vi "RootBLE.vi"() -> ()   [LabVIEW 2019]
uses:
  <userlib>/MicroPython/VIs/uPythonX/uPythonX.xctl
panel:
  in  "PyBD 3":T1(xcontrol)={"Port"="pyboard - ASRL96::INSTR", "All Code"="import bluetooth, machine, utime,ubinascii\n\ndef ble_cb(event, data):\n     global bt_event,bt_data,devices\n     bt_event = event, data\n     print('ble event:', event, data)\n     \nbt = bluetooth.Bluetooth()\nbt.active(1)\nbt_event=None\nbt.irq(ble_cb, 0xffff)\n\ndef sync_cmd(f, args, timeout_ms=1000):\n    global bt_event\n    event = []\n    bt_event = None # clear event\n    f(*args) # call function\n    t0 = utime.ticks_ms()\n    while time.ticks_diff(time.ticks_ms(), t0) < timeout_ms:\n        if bt_event is not None:\n             event.append(bt_event)\n             bt_event = None\n        machine.idle() \n    return event\n    #raise OSError('timeout')\n\n# use it like this\nread_result = sync_cmd(bt.scan, (5000), 5000)\nfor i in read_result:\n     print('Addr type: %d mac addr: %s'%(i[1][0],ubinascii.hexlify(i[1][1],':')))\n\nsync_cmd(bt.connect,(1,b'\\x34\\x15\\x13\\x7F\\xD5\\xCC'))\n\n#bt.connect(2,b'\\x34\\x15\\x13\\x7F\\xD5\\xCC')"}
  in  "VISA resource name":refnum<visa-resource-name>
  in  "PyBD 2":T1(xcontrol)={"Port"="PyBoard - ASRL44::INSTR", "All Code"="import bluetooth, machine, utime\n\nbt_event = 0,0\nbt_data = []\ndevices = []\n\ndef ble_cb(event, data):\n     global bt_event,bt_data,devices\n     bt_event = event, data\n     if event == 16:\n          devices.append(data)\n     else:\n          bt_data.append(bt_event)\n     print('ble event:', event, data)\n          \n\nbt = bluetooth.Bluetooth()\nbt.active(1)\nbt_event=None\nbt.irq(ble_cb, 0xffff)\n\n\nbt.connect(1,b'\\xf6\\x1d\\xa5\\xe2^\\xf5')\n\nbt.disconnect(64)\n\nwhile not bt_event:\n     machine.idle()\n\nbt.gattc_write(14, 64, b'\\x01')\n\n'''\nThen the available functions for central mode are:\n\nbt.connect(addr_type, mac, scan_duration_ms=2000)\nbt.scan(duration_ms)\nbt.gattc_disc_svcs(conn_handle)\nbt.gattc_disc_chrs(start_handle, end_handle, conn_handle)\nbt.gattc_disc_dscs(start_handle, end_handle, conn_handle)\nbt.gattc_read(value_handle, conn_handle)\nbt.gattc_write(value_handle, conn_handle, data)\n\nUsually conn_handle would be 64.  addr_type should probably be 0 (or maybe 2).  mac should be the MAC address of the root robot, which can be found by doing a scan (results come in through the ble_cb callback).\n\nYou then need to find the value handles for the tx/rx characteristics on the root robot.  This is done using: bt.gattc_disc_chrs(0, 0xffff, 64).  ble_cb will then be called with the results of this discovery process and the returned data will include the tx/rx uuid along with the value handle for it (but I'm not sure exactly of the format of the returned data for this...).\n\n'''\nbt_data = []\ndevices = []\nstarttime = utime.time()\nbt.scan(5000)\nwhile (utime.time()- starttime) < 5:\n     bt_event=None\n     while not bt_event:\n          machine.idle()\n     \n\nbt.connect(0, b'M\\x0b\\xf0\\xf9\\x81\\x00')\n\n# ble event: 16 (1, b'\\xf6\\x1d\\xa5\\xe2^\\xf5', True, 198, b'\\x02\\x01\\x06\\x11\\x06yI\\xb0\"\\x98\\x0c\\xa3\\x97-D*\\xac(\\xd8\\xc5H')\nbt.connect(1,b'\\xf6\\x1d\\xa5\\xe2^\\xf5')\n#ble event: 64 (1, b'\\xf6\\x1d\\xa5\\xe2^\\xf5', 64)\nbt.gattc_disc_svcs(64)\n'''\nble event: 256 (1, 7, UUID16(0x1800), 64)\nble event: 256 (8, 8, UUID16(0x1801), 64)\nble event: 256 (9, 14, UUID128('6e400001-b5a3-f393-e0a9-e50e24dcca9e'), 64)\nble event: 256 (15, 30, UUID16(0x180a), 64)\nble event: 256 (31, 65535, UUID128('48c5d828-ac2a-442d-97a3-0c9822b04979'), 64)\n     \nble event: 256 (64, 1, 7, UUID16(0x1800))\nble event: 256 (64, 8, 8, UUID16(0x1801))\nble event: 256 (64, 9, 14, UUID128('9ecadc24-0ee5-a9e0-93f3a3b50100406e')) # uart_identifier_uuid\nble event: 256 (64, 15, 30, UUID16(0x180a))\nble event: 256 (64, 31, 65535, UUID128('7949b022-980c-a397-2d442aac28d8c548'))  # root_identifier_uuid - backwards\n'''\n#bt.gattc_discover_characteristics(64, 9, 14)\n\n\nbt.gattc_disc_chrs(9,14,64)\nbt.gattc_disc_chrs(1,7,64)\nbt.gattc_read(3,64)   # get name\nbt.gattc_disc_dscs(1, 65535, 64)\nbt.gattc_write(14, 64, b'\\x01')\n\ndef get_name (data):\n     bt.connect(data[0],data[1])\n     bt.data=[]\n     whilin\n     bt.gattc_disc_svcs(64)\n     bt.gattc_disc_chrs(9,14,64)\n     \n\n'''\n1. get listing of all BT devices\n2. connect to each and\n3. ask for all servies\n4. find service 0x1800 - discover characteristics\n5. do a read of the characterstic for 0x2A00\n6. take the last (3rd) element - that is the name\n7. disconnect\n'''\nble event: 512 (10, 11, 12, UUID128('6e400002-b5a3-f393-e0a9-e50e24dcca9e'), 64)\nble event: 512 (12, 13, 16, UUID128('6e400003-b5a3-f393-e0a9-e50e24dcca9e'), 64)\n     \n\nble event: 512 (64, 10, 11, 12, UUID128('9ecadc24-0ee5-a9e0-93f3a3b50200406e'))   #  tx characteristic\nble event: 512 (64, 12, 13, 16, UUID128('9ecadc24-0ee5-a9e0-93f3a3b50300406e'))   #  rx characteristic\n'''\nforward = [0x01, 0x04, 0x00, 0x00, 0x00, 0x00, 0x64, 0x00, 0x00, 0x00, 0x64, 0x00, 0x00, 0x00, 0x00, 0x00, 0x00, 0x00, 0x00, 0xD1]\nleft = [0x01, 0x04, 0x00, 0x00, 0x00, 0x00, 0x00, 0x00, 0x00, 0x00, 0x64, 0x00, 0x00, 0x00, 0x00, 0x00, 0x00, 0x00, 0x00, 0x8A]\nright = [0x01, 0x04, 0x00, 0x00, 0x00, 0x00, 0x64, 0x00, 0x00, 0x00, 0x00, 0x00, 0x00, 0x00, 0x00, 0x00, 0x00, 0x00, 0x00, 0x25]\nstop = [0x01, 0x04, 0x00, 0x00, 0x00, 0x00, 0x00, 0x00, 0x00, 0x00, 0x00, 0x00, 0x00, 0x00, 0x00, 0x00, 0x00, 0x00, 0x00, 0x7E]\nbackwards = [0x01, 0x04, 0x00, 0xFF, 0xFF, 0xFF, 0x9C, 0xFF, 0xFF, 0xFF, 0x9C, 0x00, 0x00, 0x00, 0x00, 0x00, 0x00, 0x00, 0x00, 0x71]\npen_up = [0x02, 0x00, 0x00, 0x00, 0x00, 0x00, 0x00, 0x00, 0x00, 0x00, 0x00, 0x00, 0x00, 0x00, 0x00, 0x00, 0x00, 0x00, 0x00, 0x00]\npen_down = [0x02, 0x00, 0x00, 0x01, 0x00, 0x00, 0x00, 0x00, 0x00, 0x00, 0x00, 0x00, 0x00, 0x00, 0x00, 0x00, 0x00, 0x00, 0x00, 0x00]\n\nbt.gattc_write(11, 64, bytearray(pen_down))\n\n\n\nbt.gattc_read(16,64)\n# ble event: 2048 (16, 64, b'\\x02\\x11\\x00%*')\n\nbt.disconnect(64)\n\n\ndef TranslateMessage(data):\n     type = ''\n     if event == 2048:\n          message = data[2][0]\n          if message == 4:\n               type = 'Color Sensor'\n          elif message == 12:\n               type = 'Bumper'\n          elif message == 13:\n               type = 'Light Sensor'\n          elif message == 17:\n               type = 'Touch Sensor'\n          elif message == 20:\n               type = 'Cliff Sensor'\n          print(type, message)\n          return data\n          \n'''\n\u0016ble event: 8192 (13, 64, b'\\x11\\x00\\x00\\x00\\x03\\x1dC@\\x00\\x00\\x00\\x00\\x00\\x00\\x00\\x00\\x00\\x00\\x00\\x17')\nble event: 8192 (13, 64, b'\\x11\\x00\\x01\\x00\\x03\\x1d\\xd9\\x00\\x00\\x00\\x00\\x00\\x00\\x00\\x00\\x00\\x00\\x00\\x00!')\nble event: 8192 (13, 64, b'\\r\\x00\\x02\\x00\\x03\\x1e\\xd4\\x06\\x02\\x13\\x00\\x7f\\x00\\x00\\x00\\x00\\x00\\x00\\x00d')\nble event: 8192 (13, 64, b'\\x11\\x00\\x03\\x00\\x03$\\x19@\\x00\\x00\\x00\\x00\\x00\\x00\\x00\\x00\\x00\\x00\\x00D')\nble event: 8192 (13, 64, b'\\x11\\x00\\x04\\x00\\x03%w\\x00\\x00\\x00\\x00\\x00\\x00\\x00\\x00\\x00\\x00\\x00\\x00f')\nble event: 8192 (13, 64, b'\\x0c\\x00\\x05\\x00\\x03*#@\\x00\\x00\\x00\\x00\\x00\\x00\\x00\\x00\\x00\\x00\\x00y')\nble event: 8192 (13, 64, b'\\x0c\\x00\\x06\\x00\\x03+\\x9a\\x00\\x00\\x00\\x00\\x00\\x00\\x00\\x00\\x00\\x00\\x00\\x00\\xf3')\nble event: 8192 (13, 64, b'\\x0c\\x00\\x07\\x00\\x031|\\x80\\x00\\x00\\x00\\x00\\x00\\x00\\x00\\x00\\x00\\x00\\x00\\xb8')\nble event: 8192 (13, 64, b'\\x0c\\x00\\x08\\x00\\x036\\x91\\x00\\x00\\x00\\x00\\x00\\x00\\x00\\x00\\x00\\x00\\x00\\x00\\x9f')\nble event: 8192 (13, 64, b'\\x11\\x00\\t\\x00\\x03A\\x87\\x80\\x00\\x00\\x00\\x00\\x00\\x00\\x00\\x00\\x00\\x00\\x00g')\nble event: 8192 (13, 64, b'\\x11\\x00\\n\\x00\\x03C\\xdf\\x00\\x00\\x00\\x00\\x00\\x00\\x00\\x00\\x00\\x00\\x00\\x00\\xca')\nble event: 8192 (13, 64, b'\\x11\\x00\\x0b\\x00\\x03DC\\x80\\x00\\x00\\x00\\x00\\x00\\x00\\x00\\x00\\x00\\x00\\x00W')\nble event: 8192 (13, 64, b'\\x11\\x00\\x0c\\x00\\x03D\\xd9\\x00\\x00\\x00\\x00\\x00\\x00\\x00\\x00\\x00\\x00\\x00\\x00*')\nble event: 8192 (13, 64, b'\\x11\\x00\\r\\x00\\x03H]@\\x00\\x00\\x00\\x00\\x00\\x00\\x00\\x00\\x00\\x00\\x00\\x0e')\nble event: 8192 (13, 64, b'\\x11\\x00\\x0e\\x00\\x03IW\\x00\\x00\\x00\\x00\\x00\\x00\\x00\\x00\\x00\\x00\\x00\\x00O')\nble event: 8192 (13, 64, b'\\x11\\x00\\x0f\\x00\\x03K\\xe1 \\x00\\x00\\x00\\x00\\x00\\x00\\x00\\x00\\x00\\x00\\x00\\x1c')\nble event: 8192 (13, 64, b'\\x11\\x00\\x10\\x00\\x03Lw\\x00\\x00\\x00\\x00\\x00\\x00\\x00\\x00\\x00\\x00\\x00\\x00}')\nble event: 8192 (13, 64, b'\\x14\\x00\\x11\\x00\\x03m\\xfc\\x01\\x00.\\x001\\x00\\x00\\x00\\x00\\x00\\x00\\x00\\x87')\nble event: 8192 (13, 64, b'\\r\\x00\\x12\\x00\\x03|~\\x06\\x01\\xb2\\x00x\\x00\\x00\\x00\\x00\\x00\\x00\\x00Q')\n     '''"}
  in  "Pi":T1(xcontrol)={"Port"="Spike - ASRL73::INSTR", "All Code"="#!/usr/bin/env python3\n# https://github.com/zlite/PyRoot/blob/master/drive-root.py\n\nimport gatt\nimport threading\nimport time,termios,tty,sys\n\ninstructions = \"\"\"---------------------\n KEY         COMMAND\n---------------------\n w           Forward\n s           Backward\n a           Left\n d           Right\n space       Stop\n t           Turn\n o           Pen Up\n l           Pen Down\n q           Quit\"\"\"\n\n# BLE UUID's\nroot_identifier_uuid = '48c5d828-ac2a-442d-97a3-0c9822b04979'\nuart_service_uuid = '6e400001-b5a3-f393-e0a9-e50e24dcca9e'\ntx_characteristic_uuid = '6e400002-b5a3-f393-e0a9-e50e24dcca9e' # Write\nrx_characteristic_uuid = '6e400003-b5a3-f393-e0a9-e50e24dcca9e' # Notify\n\nclass BluetoothDeviceManager(gatt.DeviceManager):\n    robot = None # root robot device\n\n    def device_discovered(self, device):\n        print(\"[%s] Discovered: %s\" % (device.mac_address, device.alias()))\n        self.stop_discovery() # Stop searching\n        self.robot = RootDevice(mac_address=device.mac_address, manager=self)\n        self.robot.connect()\n\nclass RootDevice(gatt.Device):\n    def connect_succeeded(self):\n        super().connect_succeeded()\n        print(\"[%s] Connected\" % (self.mac_address))\n\n    def connect_failed(self, error):\n        super().connect_failed(error)\n        print(\"[%s] Connection failed: %s\" % (self.mac_address, str(error)))\n\n    def disconnect_succeeded(self):\n        super().disconnect_succeeded()\n        print(\"[%s] Disconnected\" % (self.mac_address))\n\n    def services_resolved(self):\n        super().services_resolved()\n        print(\"[%s] Resolved services\" % (self.mac_address))\n\n        self.uart_service = next(\n            s for s in self.services\n            if s.uuid == uart_service_uuid)\n\n        self.tx_characteristic = next(\n            c for c in self.uart_service.characteristics\n            if c.uuid == tx_characteristic_uuid)\n\n        self.rx_characteristic = next(\n            c for c in self.uart_service.characteristics\n            if c.uuid == rx_characteristic_uuid)\n\n        self.rx_characteristic.enable_notifications() # listen to RX messages\n\n    def characteristic_value_updated(self, characteristic, value):\n        message = []\n        type = \"\"\n        for byte in value:\n            message.append(byte)\n#        print (\"Messages from Root:\")\n        if message[0] == 4: type = \"Color Sensor\"\n        if message[0] == 12: type = \"Bumper\"\n        if message[0] == 13: type = \"Light Sensor\"\n        if message[0] == 17: type = \"Touch Sensor\"\n        if message[0] == 20: type = \"Cliff Sensor\"\n\n        print(type, message)\n\n    def drive_forward(self):\n        self.tx_characteristic.write_value([0x01, 0x04, 0x00, 0x00, 0x00, 0x00, 0x64, \n0x00, 0x00, 0x00, 0x64, 0x00, 0x00, 0x00, 0x00, 0x00, 0x00, 0x00, 0x00, 0xD1])\n\n    def drive_left(self):\n        self.tx_characteristic.write_value([0x01, 0x04, 0x00, 0x00, 0x00, 0x00, 0x00, 0x00, 0x00, 0x00, 0x64, 0x00, 0x00, 0x00, 0x00, 0x00, 0x00, 0x00, 0x00, 0x8A])\n\n    def drive_right(self):\n        self.tx_characteristic.write_value([0x01, 0x04, 0x00, 0x00, 0x00, 0x00, 0x64, 0x00, 0x00, 0x00, 0x00, 0x00, 0x00, 0x00, 0x00, 0x00, 0x00, 0x00, 0x00, 0x25])\n\n    def stop(self):\n        self.tx_characteristic.write_value([0x01, 0x04, 0x00, 0x00, 0x00, 0x00, 0x00, 0x00, 0x00, 0x00, 0x00, 0x00, 0x00, 0x00, 0x00, 0x00, 0x00, 0x00, 0x00, 0x7E])\n\n    def drive_backwards(self):\n        self.tx_characteristic.write_value([0x01, 0x04, 0x00, 0xFF, 0xFF, 0xFF, 0x9C, 0xFF, 0xFF, 0xFF, 0x9C, 0x00, 0x00, 0x00, 0x00, 0x00, 0x00, 0x00, 0x00, 0x71])\n\n    def pen_up(self):\n        self.tx_characteristic.write_value([0x02, 0x00, 0x00, 0x00, 0x00, 0x00, 0x00, 0x00, 0x00, 0x00, 0x00, 0x00, 0x00, 0x00, 0x00, 0x00, 0x00, 0x00, 0x00, 0x00])\n\n    def pen_down(self):\n        self.tx_characteristic.write_value([0x02, 0x00, 0x00, 0x01, 0x00, 0x00, 0x00, 0x00, 0x00, 0x00, 0x00, 0x00, 0x00, 0x00, 0x00, 0x00, 0x00, 0x00, 0x00, 0x00])\n\n    def turn_rate(self, rate):\n        left = 0\n        right = 0\n        if rate >= 0:\n            left = rate\n        if rate < 0:\n            right = -1*rate\n        leftbytes = left.to_bytes(4,byteorder='big',signed=True)  # need to convert to byte string\n        rightbytes = right.to_bytes(4,byteorder='big',signed=True)\n        # note that we're not dynamically calculating the CRC at the end, so just leaving it 0 (unchecked)\n        self.tx_characteristic.write_value([0x01, 0x04, 0x00, leftbytes[0], leftbytes[1], leftbytes[2], leftbytes[3], rightbytes[0], rightbytes[1], rightbytes[2], rightbytes[3], 0x00, 0x00, 0x00, 0x00, 0x00, 0x00, 0x00, 0x00, 0x0])\n\n    def steer(self, left, right):\n        leftbytes = left.to_bytes(4,byteorder='big',signed=True)  # need to convert to byte string\n        rightbytes = right.to_bytes(4,byteorder='big',signed=True)\n        # note that we're not dynamically calculating the CRC at the end, so just leaving it 0 (unchecked)\n        self.tx_characteristic.write_value([0x01, 0x04, 0x00, leftbytes[0], leftbytes[1], leftbytes[2], leftbytes[3], rightbytes[0], rightbytes[1], rightbytes[2], rightbytes[3], 0x00, 0x00, 0x00, 0x00, 0x00, 0x00, 0x00, 0x00, 0x0])\n\n\ndef drive_root(command):\n    angle = 0\n    if command == \"w\":\n        print (\"Drive forward\")\n        manager.robot.drive_forward()\n    if command == \"s\":\n        print (\"Drive backwards\")\n        manager.robot.drive_backwards()\n    if command == \"d\":\n        print (\"Drive right\")\n        manager.robot.drive_right()\n    if command == \"a\":\n        print (\"Drive left\")\n        manager.robot.drive_left()\n    if command == \" \":\n        print (\"Stop\")\n        manager.robot.stop()\n    if command == \"o\":\n        print (\"Pen up\")\n        manager.robot.pen_up()\n    if command == \"l\":\n        print (\"Pen down\")\n        manager.robot.pen_down()\n    if command == \"t\":\n        print (\"Enter turn rate (up to +-90):\")\n        char = input()\n        rate = int(char)\n        print (\"Turning \", rate)\n        manager.robot.turn_rate(rate)\n    if command == \"p\":\n        print (\"Steer\")\n        manager.robot.steer(30,40)\n\n# keybaord inputs\ndef getch():\n    fd = sys.stdin.fileno()\n    old_settings = termios.tcgetattr(fd)\n    try:\n        tty.setraw(sys.stdin.fileno())\n        ch = sys.stdin.read(1)\n    finally:\n        termios.tcsetattr(fd, termios.TCSADRAIN, old_settings)\n    return ch\n\n# start here if run as program / not imported as module\nif __name__ == \"__main__\":\n    manager = BluetoothDeviceManager(adapter_name = 'hci0')\n    manager.start_discovery(service_uuids=[root_identifier_uuid])\n    thread = threading.Thread(target = manager.run)\n    thread.start()\n    char = \"\"\n    try:\n        while manager.robot is None:\n            pass # wait for a root robot to be discovered\n        print(instructions)\n        while char != \"q\":\n            char = getch() # wait for keyboard input\n            drive_root(char)\n        print(\"Quitting\")\n        manager.stop()\n        manager.robot.disconnect()\n        thread.join()\n    except KeyboardInterrupt:\n        pass"}
  in  "BLE - Root":T1(xcontrol)={"Port"="PyBoard - ASRL44::INSTR", "All Code"="import hub,utime\n# BLE UUID's\nroot_identifier_uuid = '48c5d828-ac2a-442d-97a3-0c9822b04979'\nuart_service_uuid = '6e400001-b5a3-f393-e0a9-e50e24dcca9e'\ntx_characteristic_uuid = '6e400002-b5a3-f393-e0a9-e50e24dcca9e' # Write\nrx_characteristic_uuid = '6e400003-b5a3-f393-e0a9-e50e24dcca9e' # Notify\n\ndrive_forward = [0x01, 0x04, 0x00, 0x00, 0x00, 0x00, 0x64, 0x00, 0x00, 0x00, 0x64, 0x00, 0x00, 0x00, 0x00, 0x00, 0x00, 0x00, 0x00, 0xD1]\n\nhub.ble.rssi(-70)\nhub.ble.scan(1)\nutime.sleep(1)\ndevices = hub.ble.scan_result()\n\ndesired = [x for x in devices if x['service_id'].upper() == root_identifier_uuid.upper()]\n\ndef connect_callback(a):\n     print('Connection complete: {0}'.format(a))\n\n'''desired = -1\ncounter = 0\nfor device in devices:\n     if device['service_id'] == root_identifier_uuid.upper():\n          desired = counter\n          print('found '+ str(desired))\n          print (device)\n     counter += 1\n   '''\nhub.ble.callback(connect_callback)\nroot = hub.ble.connect(desired)\n\n'''\n     root.send(drive_forward)\n     root.disconnect()\n'''"}
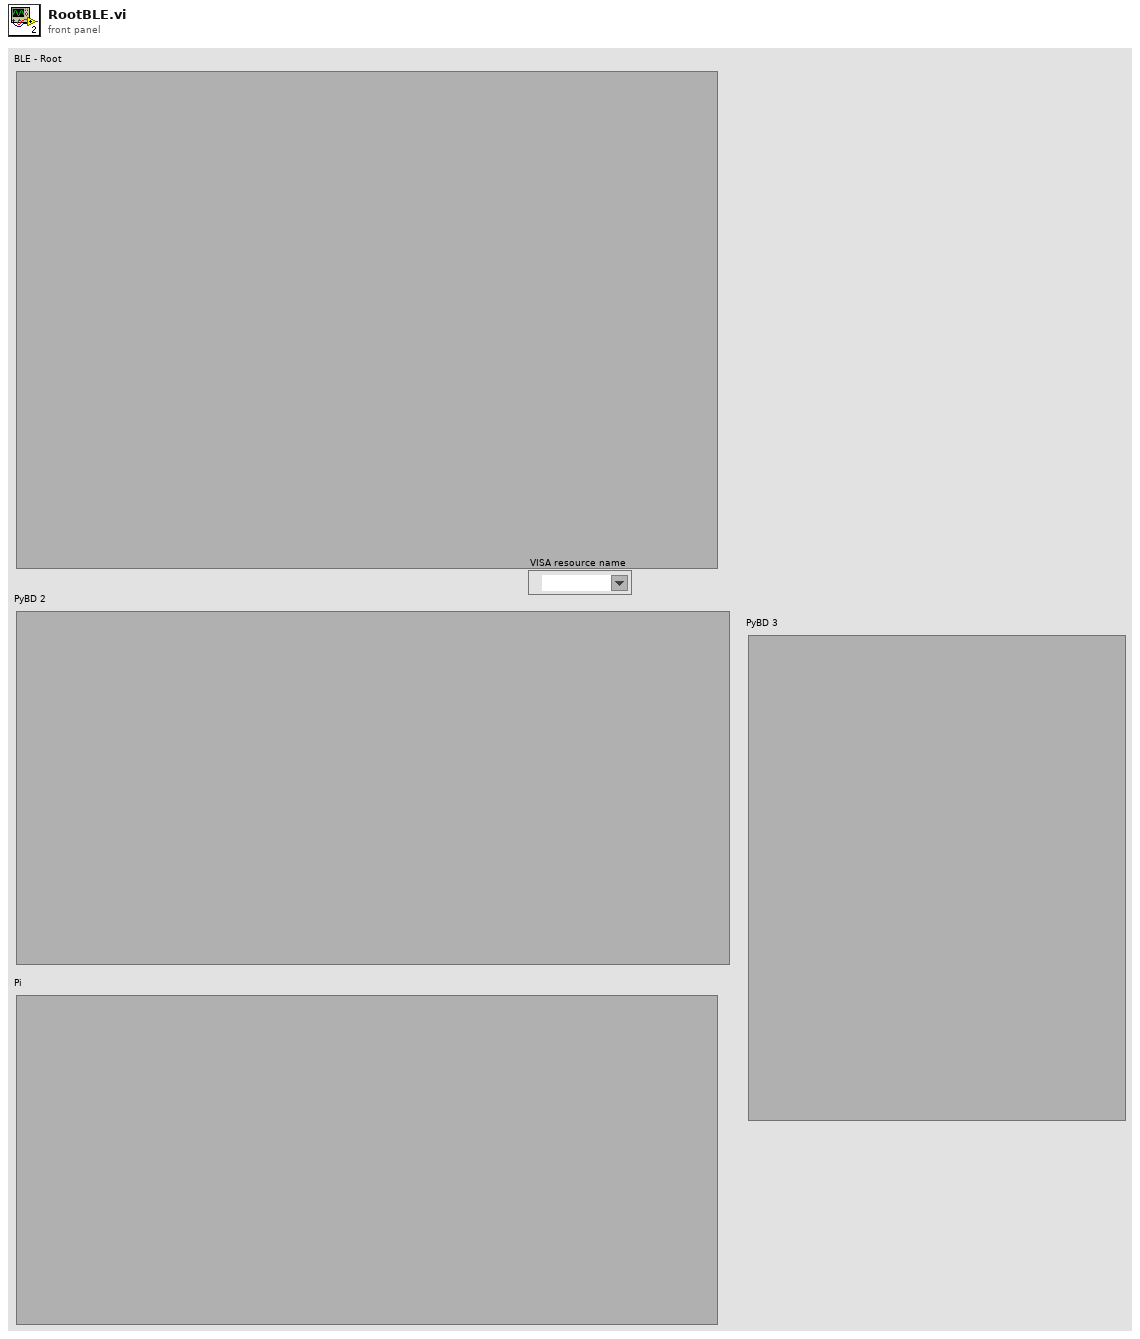
[diagram p1: front panel]
types:
  T1 = cluster{"Port":refnum<visa-resource-name>, "All Code":string}
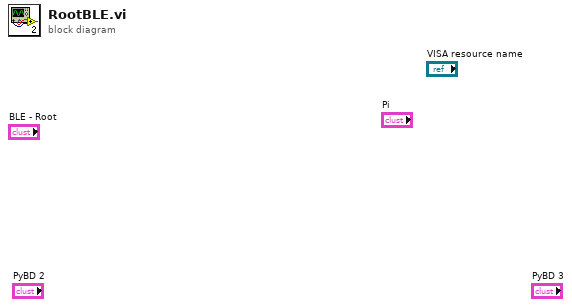
[diagram p0: block diagram]
diagram:
